vi "XPARTD_SearchRunningDisp.vi"(8 "error in (no error)":errorcluster, 9 "display":string, 10 "kill":bool) -> (0 "error out":errorcluster, 1 "any?":bool, 2 "process":i32[](array[numeric]), 3 "exists?":bool)   [LabVIEW 2016]
panel:
  out "standard output":string
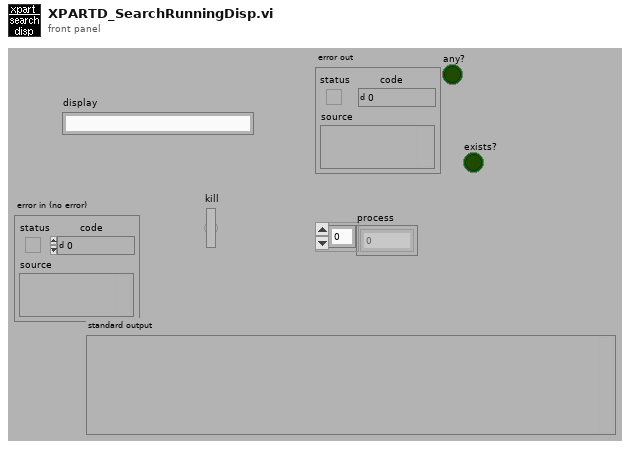
[diagram p1: front panel]
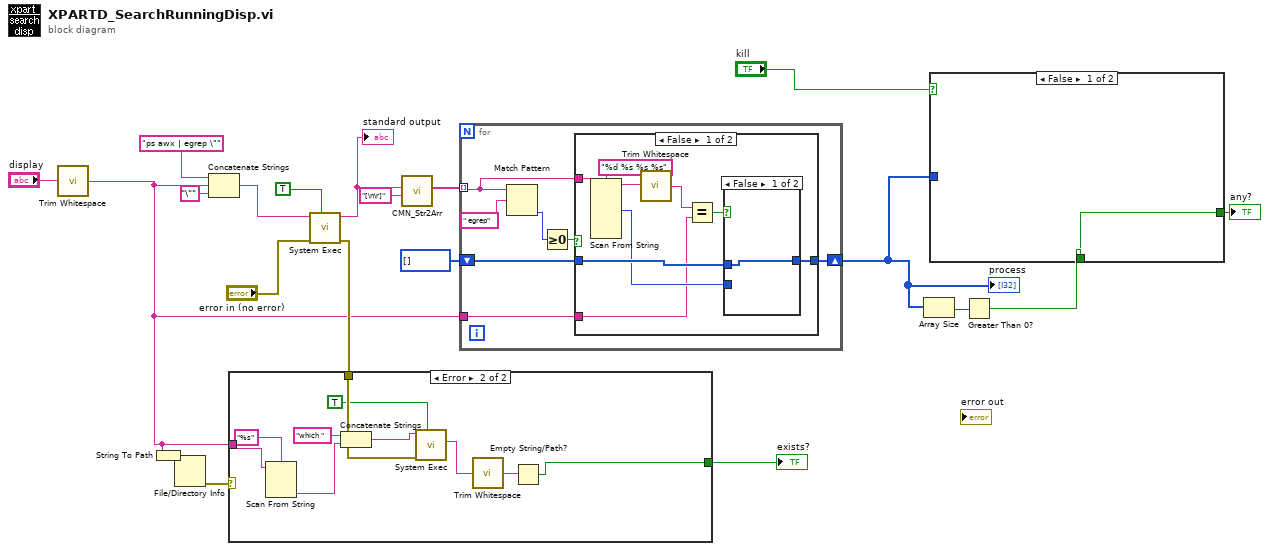
[diagram p0: block diagram]
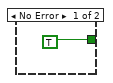
[diagram p2: hidden frame]
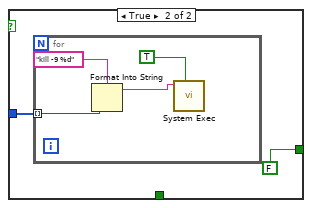
[diagram p3: hidden frame]
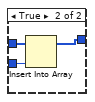
[diagram p4: hidden frame]
diagram:
  n1 = call <vilib>:"Trim Whitespace.vi"("string"="display") -> ("trimmed string"=w1:string)  [unwired: 1 in]
  n2 = String To Path(string=w1) -> (path=w4:path)
  n3 = File/Directory Info(path=w4) -> (error out=w3:errorcluster)  [unwired: 1 in, 6 out]
  n4 = Concatenate Strings("ps awx | egrep \"" ("command line"), w1, "\"" ("string")) -> (w17:string)
  n5 = call <vilib>:"System Exec.vi"("wait until completion? (T)"=TRUE, "error in (no error)"="error in (no error)", "command line"=w17) -> ("error out"=w5:errorcluster, "standard output"=w16:string)  [unwired: 3 in, 4 out]
  "standard output" <- w16
  n6 = case shown="Error" w3 {
    tunnel: w5 -> [_ w31]
    tunnel: w1 -> [_ w24]
    tunnel: [TRUE ("exists?") w25] -> w2
    frame No Error {
    }
    frame Error {
      n7 = Scan From String(format string="%s", input string=w24) -> (output 1=w22:string)  [unwired: 2 in, 4 out]
      n8 = Concatenate Strings("which " ("string"), w22) -> (w29:string)
      n9 = call <vilib>:"System Exec.vi"("wait until completion? (T)"=TRUE, "error in (no error)"=w31, "command line"=w29) -> ("standard error"=w27:string)  [unwired: 3 in, 5 out]
      n10 = call <vilib>:"Trim Whitespace.vi"("string"=w27) -> ("trimmed string"=w26:string)  [unwired: 1 in]
      n11 = Empty String/Path?(string/path=w26) -> (empty?=w25:bool)
    }
  }
  "exists?" <- w2
  n12 = call "CMN_Str2Arr.vi"("separator"="[\n\r]", "string in"=w16) -> ("Array out"=w15:string[])  [unwired: 2 in, 7 out]
  n13 = for {
    tunnel: w15 -> [w35] mode=indexing
    shift-right: [w34] -> w10
    shift-left: i32[] [] -> [w33]
    tunnel: w1 -> [w32]
    n14 = Match Pattern(string=w35, regular expression=" egrep") -> (offset past match=w37:i32)  [unwired: 4 out]
    n15 = Greater Or Equal To 0?(x=w37) -> (x >= 0?=w36:bool)
    n16 = case shown="False" w36 {
      tunnel: w35 -> [w47 _]
      tunnel: [w45 w52] -> w34
      tunnel: w33 -> [w44 w52]
      tunnel: w32 -> [w40 _]
      frame False {
        n17 = Scan From String(format string="%d %s %s %s", input string=w47) -> (remaining string=w42:string, output 1=w43:i32)  [unwired: 2 in, 9 out]
        n18 = call <vilib>:"Trim Whitespace.vi"("string"=w42) -> ("trimmed string"=w41:string)  [unwired: 1 in]
        n19 = Equal?(x=w41, y=w40) -> (x = y?=w39:bool)
        n20 = case shown="False" w39 {
          tunnel: [w48 w51] -> w45
          tunnel: w44 -> [w48 w50]
          tunnel: w43 -> [_ w49]
          frame False {
          }
          frame True {
            n21 = Insert Into Array(array=w50, new element=w49) -> (w51:i32[])  [unwired: 1 in]
          }
        }
      }
      frame True {
      }
    }
  }
  "process" <- w10
  n22 = Array Size(array=w10) -> (size(s)=w12:i32)
  n23 = Greater Than 0?(x=w12) -> (x > 0?=w7:bool)
  n24 = case shown="False" "kill" {
    tunnel: w10 -> [_ w55]
    tunnel: w7 -> [w53 _]
    tunnel: [w53 FALSE] -> w6
    frame False {
    }
    frame True {
      n25 = for {
        tunnel: w55 -> [w59] mode=indexing
        n26 = Format Into String(format string="kill -9 %d", w59) -> (resulting string=w57:string)  [unwired: 2 in, 1 out]
        n27 = call <vilib>:"System Exec.vi"("wait until completion? (T)"=TRUE, "command line"=w57) -> ()  [unwired: 4 in, 6 out]
      }
    }
  }
  "any?" <- w6
